vi "testMsgDetailsToJSON.vi"(8 "error in (no error)":errorcluster) -> (0 "error out":errorcluster)   [LabVIEW 2018]
doc: "Test the msgDetailsToJSON.vi."
uses:
  src/TcpServerBase/TcpServerBase.lvclass
  src/TcpServerBase/typedef/msgTypeDef.ctl
  <vilib>/addons/_JKI Toolkits/Caraya/classes/Assert/Assert Equal Value_Variant.vi
  <vilib>/addons/_JKI Toolkits/Caraya/classes/Test/Test.lvclass
  <vilib>/addons/_JKI Toolkits/Caraya/classes/Assert/Assert.lvclass
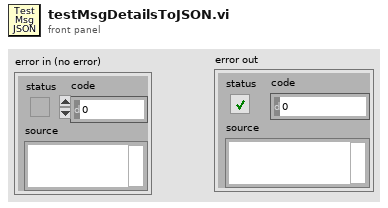
[diagram p1: front panel]
types:
  T1 = typedef "TcpServerBase.lvclass/msgTypeDef.ctl" = cluster{"msgName":string, "msgDetails":string}
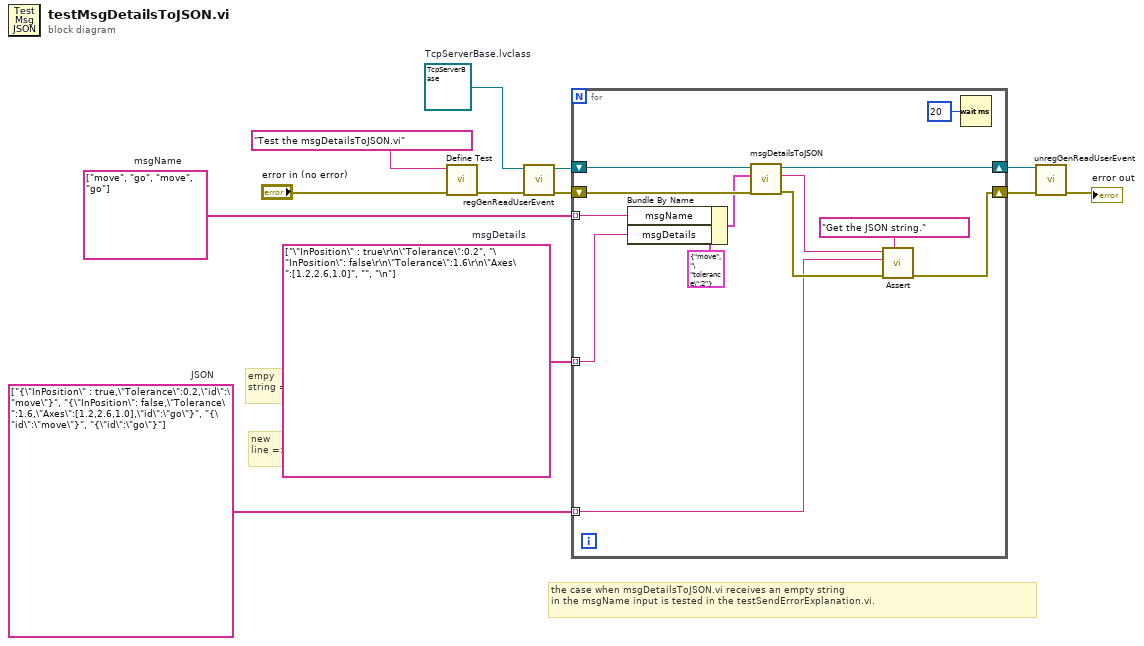
[diagram p0: block diagram]
diagram:
  w4 = refnum<class "TcpServerBase.lvclass"> refnum  # TcpServerBase.lvclass
  w8 = string[] ["{\"InPosition\" : true,\"Tolerance\":0.2,\"id\":\"move\"}", "{\"InPosition\": false,\"Tolerance\":1.6,\"Axes\":[1.2,2.6,1.0],\"id\":\"go\"}", "{\"id\":\"move\"}", "{\"id\":\"go\"}"]  # JSON
  w9 = string[] ["\"InPosition\" : true\r\n\"Tolerance\":0.2", "\"InPosition\": false\r\n\"Tolerance\":1.6\r\n\"Axes\":[1.2,2.6,1.0]", "", "\n"]  # msgDetails
  w10 = string[] ["move", "go", "move", "go"]  # msgName
  # "the case when msgDetailsToJSON.vi receives an empty string\nin the msgName input is tested in the testSendErrorExplanation.vi."
  # "new \nline =>"
  # "empy \nstring =>"
  n1 = call <vilib>:"Define Test.vi"("error in (no error)"="error in (no error)", "Label (VI Title)"="Test the msgDetailsToJSON.vi") -> ("error out"=w6:errorcluster)  [unwired: 9 in]
  n2 = call "regGenReadUserEvent.vi"("error in (no error)"=w6, "TcpServerBase in"=w4) -> ("error out"=w5:errorcluster, "TcpServerBase out"=w3:refnum<class "TcpServerBase.lvclass">)  [unwired: 8 in]
  n3 = for {
    tunnel: w10 -> [w15] mode=indexing
    tunnel: w9 -> [w14] mode=indexing
    tunnel: w8 -> [w17] mode=indexing
    shift-right: [w18] -> w7
    shift-left: w5 -> [w24]
    shift-right: [w20] -> w1
    shift-left: w3 -> [w25]
    n4 = Bundle By Name(cluster=T1 {"msgName"="move", "msgDetails"="\"tolerance\":2"} ("msgTypeDef"), "msgName"=w15, "msgDetails"=w14) -> (w13:T1)
    n5 = call "msgDetailsToJSON.vi"("error in (no error)"=w24, "msgData"=w13, "TcpServerBase in"=w25) -> ("error out"=w19:errorcluster, "JSON string"=w21:string, "TcpServerBase out"=w20:refnum<class "TcpServerBase.lvclass">)  [unwired: 6 in]
    n6 = call-poly <vilib>:"Assert.vi"("Label"="Get the JSON string.", "error in (no error)"=w19, "Y"=w17, "X"=w21) -> ("error out"=w18:errorcluster)  [unwired: 7 in]
    n7 = Wait (ms)(milliseconds to wait=u32 20) -> ()  [unwired: 1 out]
  }
  n8 = call "unregGenReadUserEvent.vi"("error in (no error)"=w7, "tcpServerBase in"=w1) -> ("error out"=→"error out":errorcluster)  [unwired: 8 in, 1 out]
